vi "Module - MQTT Server.vi"(8 "error in (no error)":errorcluster) -> (0 "error out":errorcluster)   [LabVIEW 2020]
uses:
  Control/State - MQTT Server.ctl
  <vilib>/G Open Source Project for LabVIEW/MQTT Broker/Server class/Server.lvclass
  C:/Program Files (x86)/National Instruments/LabVIEW 2020/vi.lib/LabVIEW Open Source Project/MQTT Connection/MQTT_Base/Base Class/MQTT_Base.lvclass
  <vilib>/G Open Source Project for LabVIEW/MQTT Broker/Server class/Public Events -- cluster.ctl
  Shared/Control/State - eFGV.ctl
  Control/Config File Section List.ctl
  <vilib>/G Open Source Project for LabVIEW/MQTT Broker/Server class/Server.lvclass/Server.ctl
  <vilib>/LabVIEW Open Source Project/MQTT TCP Connection/MQTT_TCP/Connection/TCPConnection.lvclass
  C:/Program Files (x86)/National Instruments/LabVIEW 2020/vi.lib/LabVIEW Open Source Project/MQTT Connection/MQTT_Connection/Connection/Connection.lvclass
  <vilib>/LabVIEW Open Source Project/MQTT Connection/MQTT_Base/Base Class/MQTT_Base.lvclass
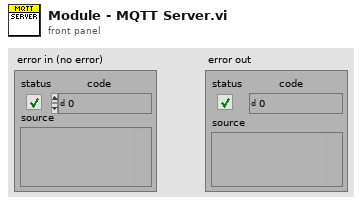
[diagram p1: front panel]
types:
  T1 = cluster{"MQTT Event":refnum<event-registration>, "User Event":refnum<event-registration>}
  T2 = cluster{"TOut":i32, "Module Name":string, "Server":refnum<class "Server.lvclass">, "User Exit":bool}
  T3 = typedef "State - MQTT Server.ctl" = enum16{"Init module", "Register for event", "Idle", "Create MQTT Broker", "Register MQTT Events", "Start MQTT Broker", "Re trigger MQTT Topic", "Stop MQTT Broker", "Unregister user event", "Close module"}
  T4 = typedef "State - eFGV.ctl" = enum16{"Init", "Read", "Write", "Close"}
  T5 = typedef "Config File Section List.ctl" = enum16{"sbRIO Setting", "RESTFUL Setting", "SQL Setting", "OPC Server Setting", "OPC Client Setting", "MQTT Server Setting", "MQTT Client Setting"}
  T6 = typedef "MQTT Server.lvlib/Server.lvclass/Public Events -- cluster.ctl" = cluster{"NbConnections":refnum<user-event>}
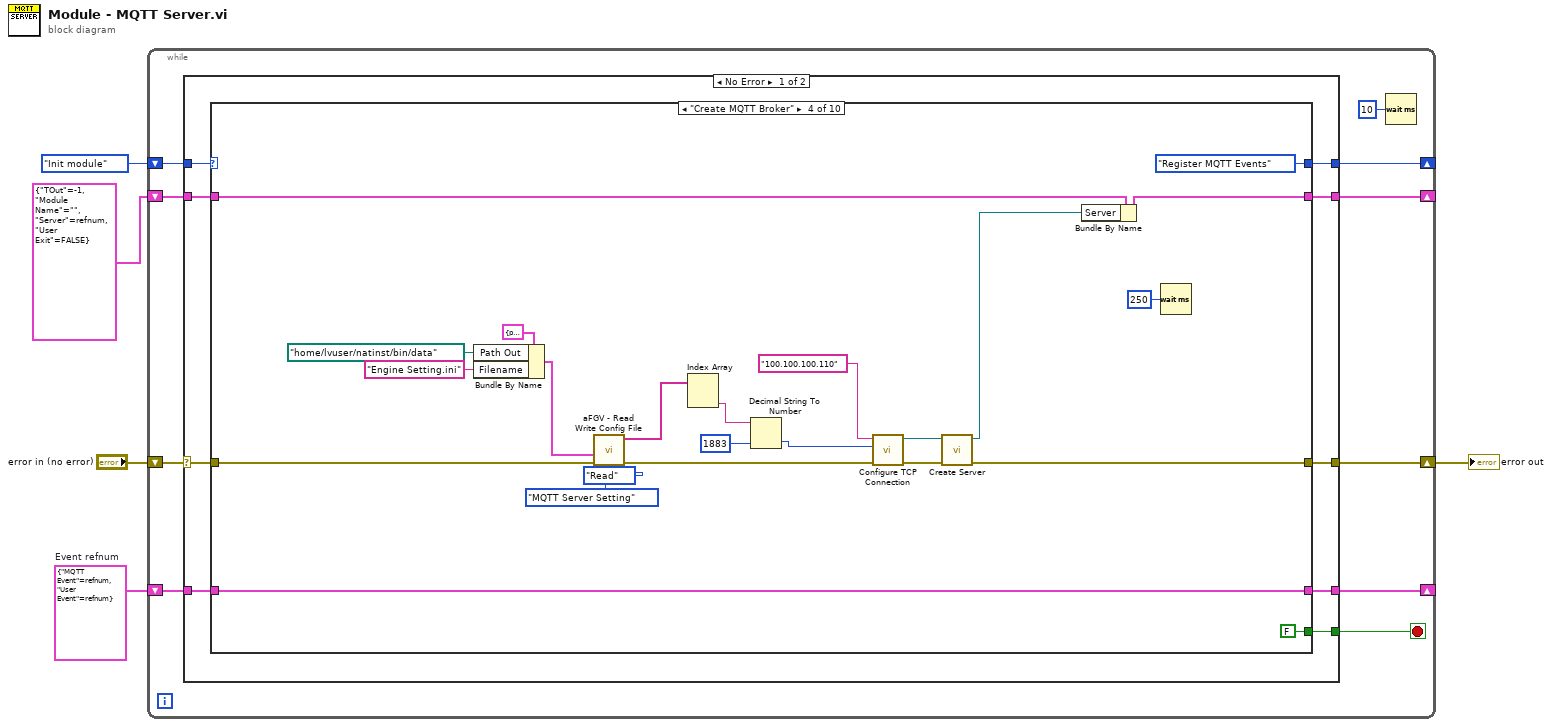
[diagram p0: block diagram]
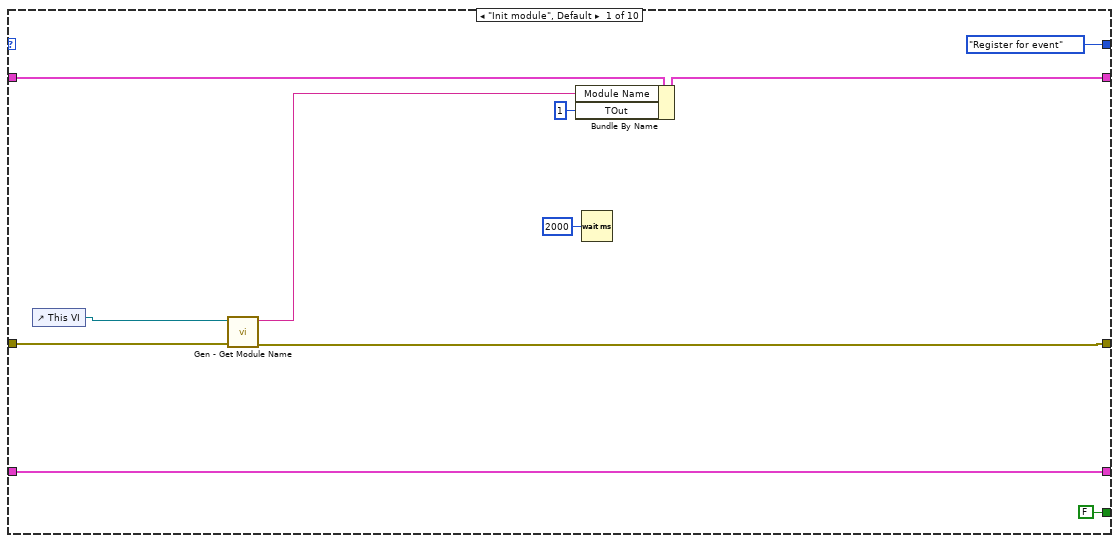
[diagram p2: hidden frame]
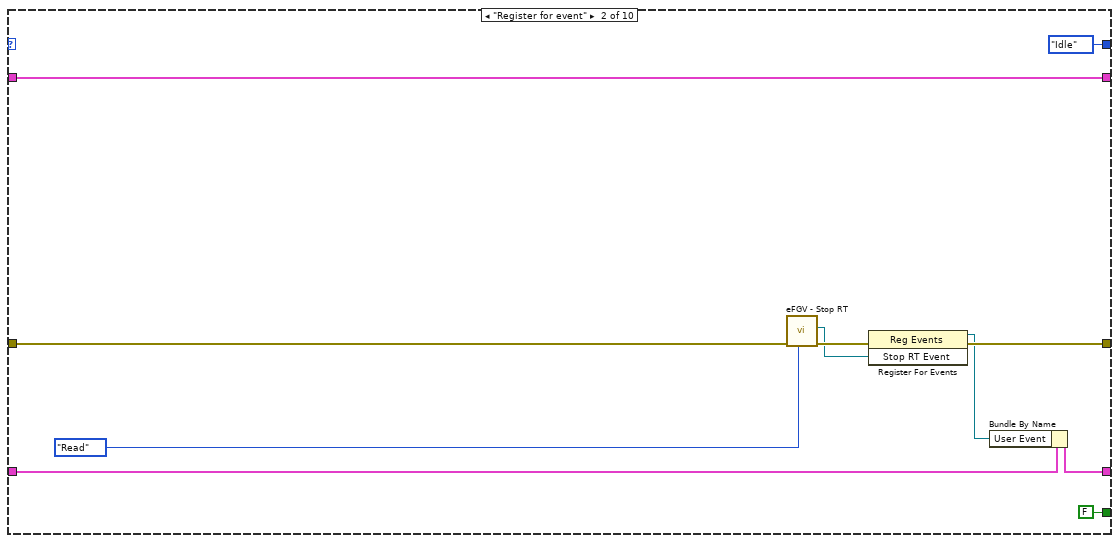
[diagram p3: hidden frame]
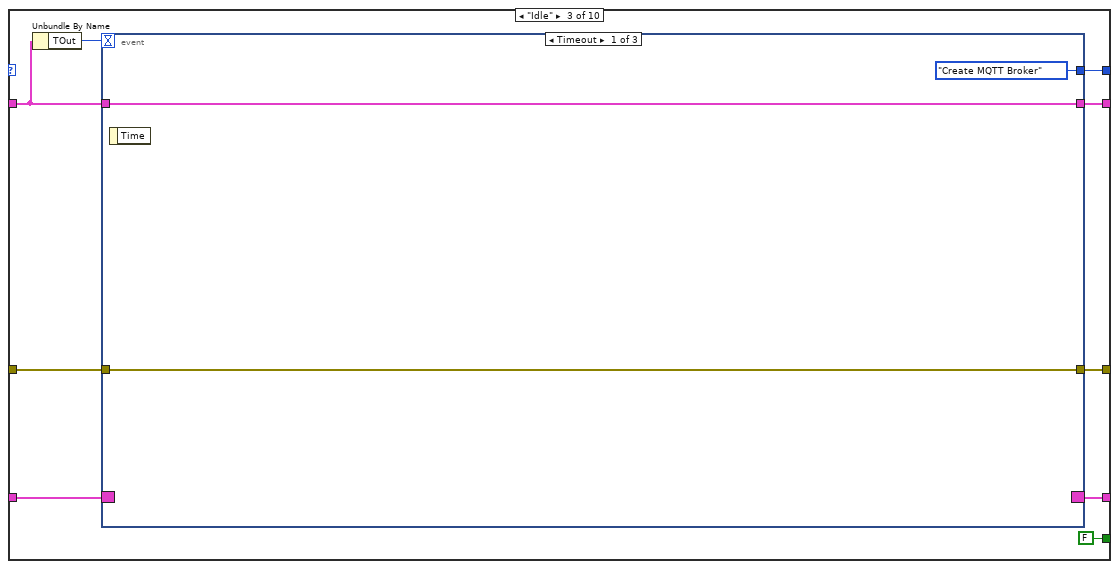
[diagram p4: hidden frame]
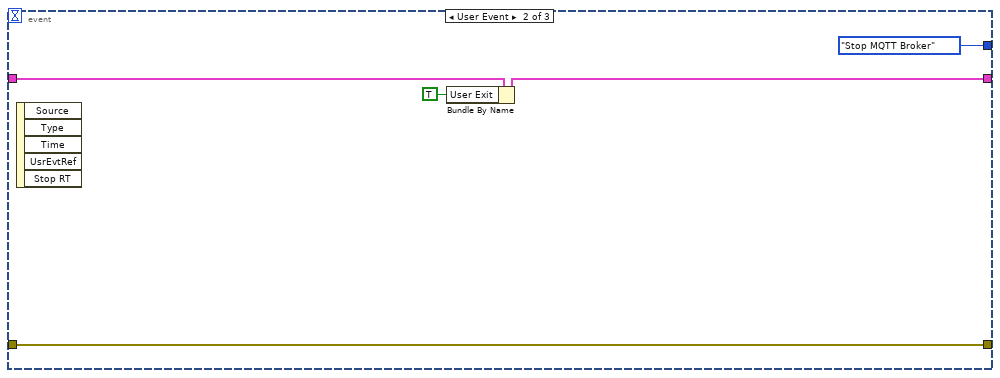
[diagram p5: hidden frame]
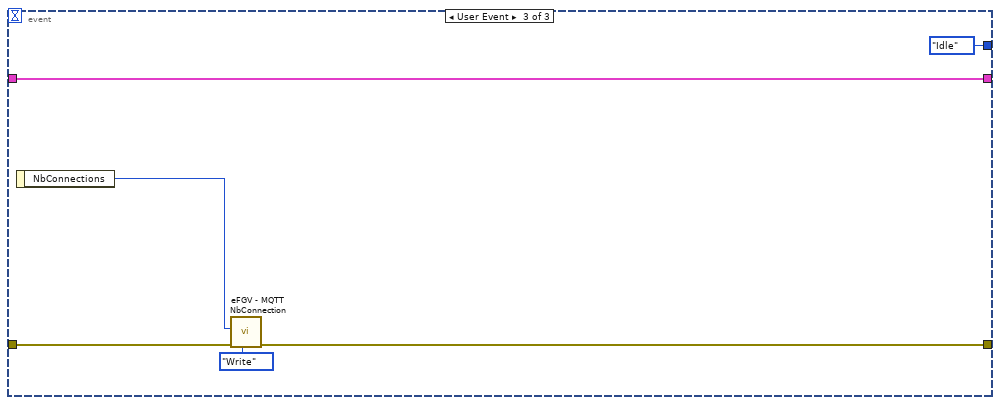
[diagram p6: hidden frame]
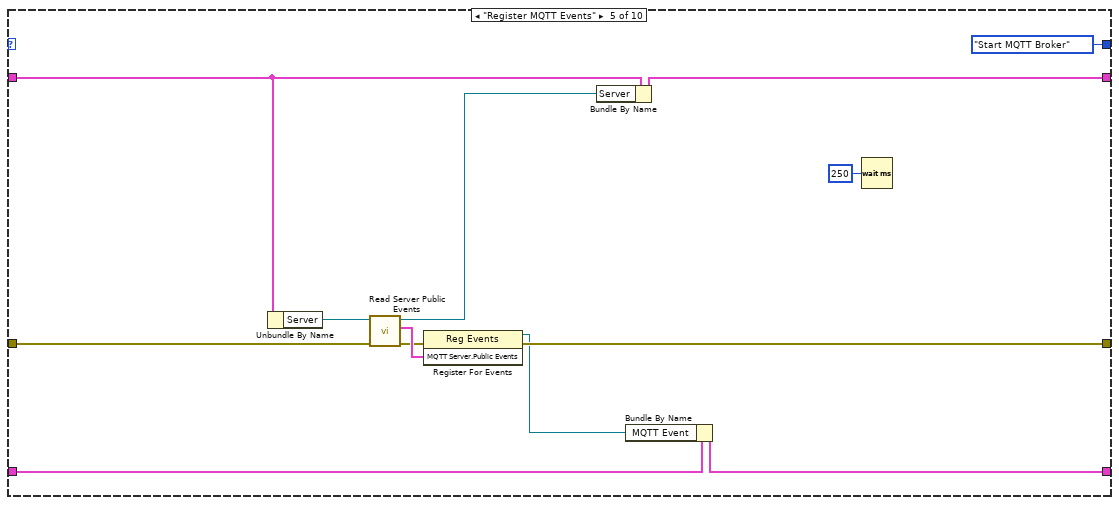
[diagram p7: hidden frame]
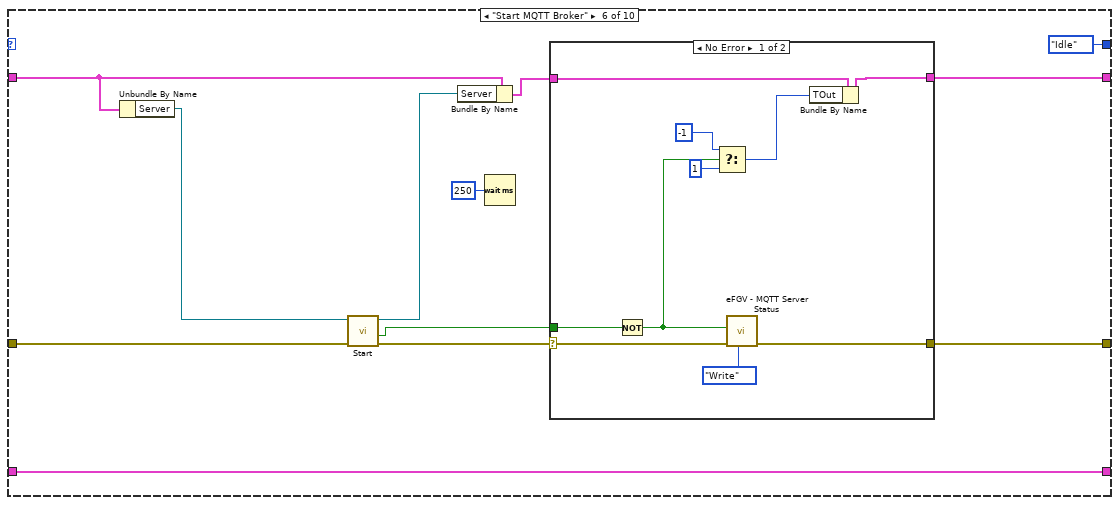
[diagram p8: hidden frame]
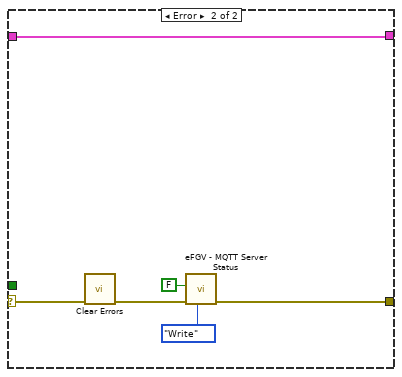
[diagram p9: hidden frame]
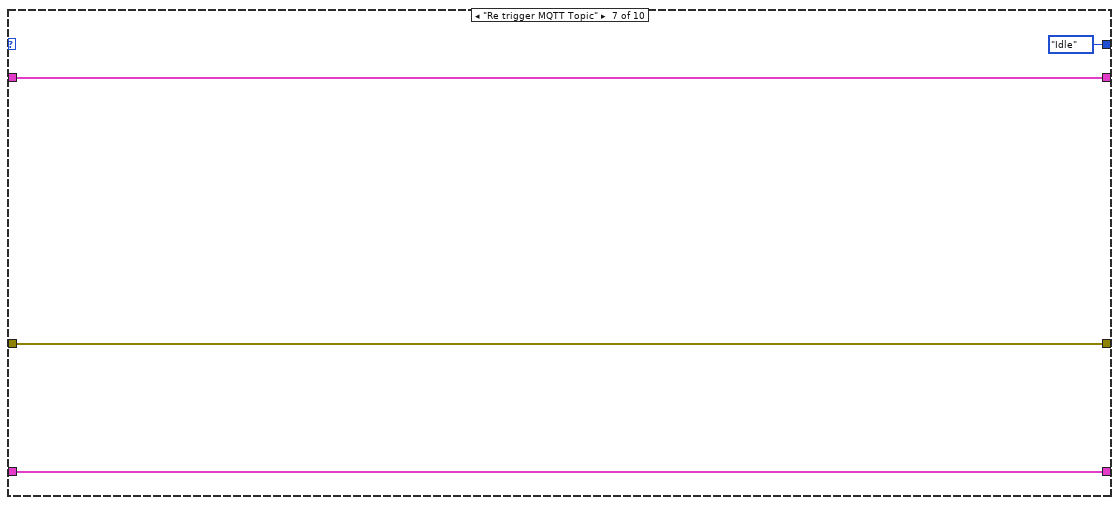
[diagram p10: hidden frame]
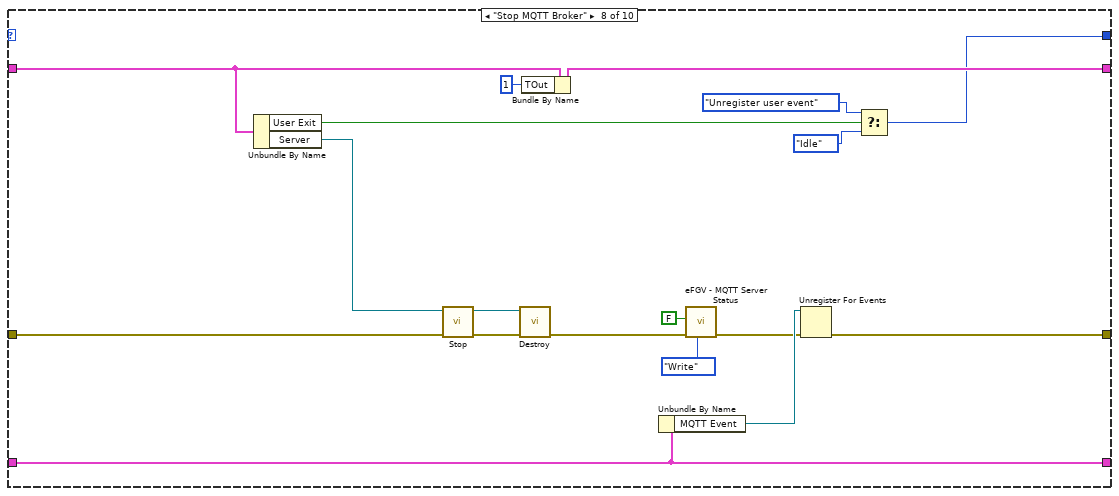
[diagram p11: hidden frame]
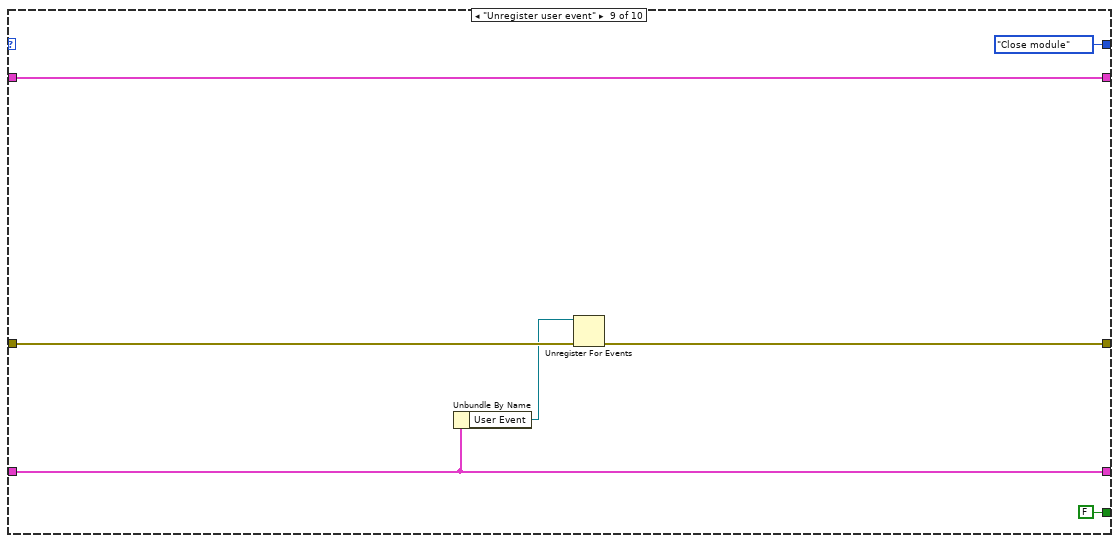
[diagram p12: hidden frame]
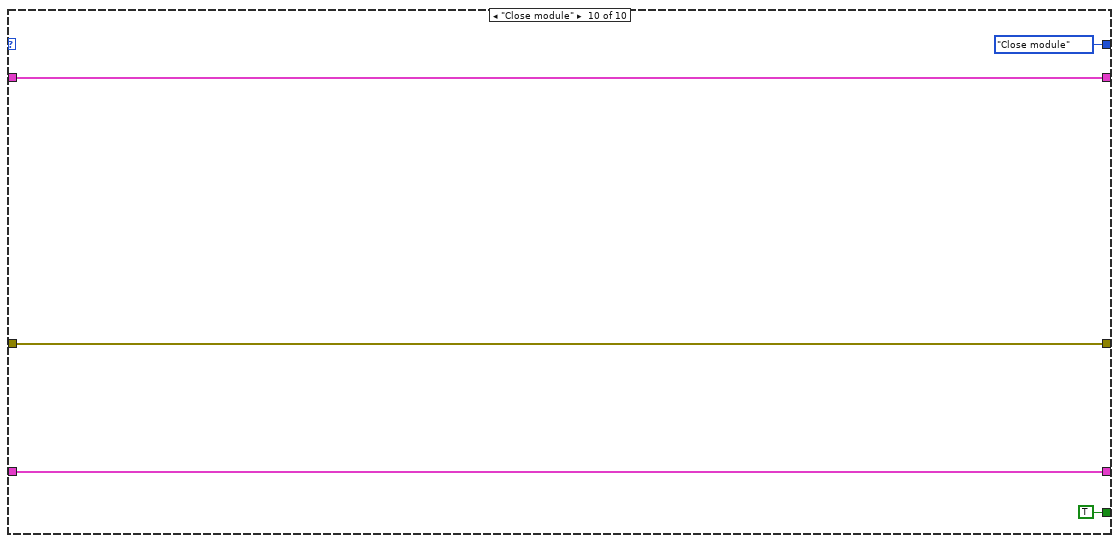
[diagram p13: hidden frame]
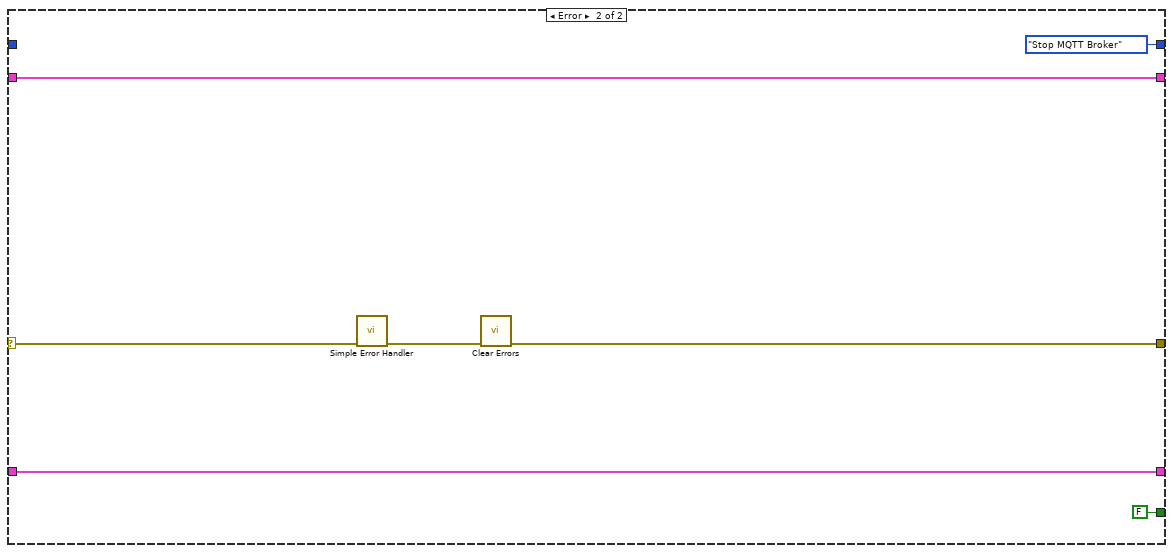
[diagram p14: hidden frame]
diagram:
  w1 = T1 {"MQTT Event"=refnum, "User Event"=refnum}  # Event refnum
  n1 = while {
    shift-right: [w11] -> w4
    shift-left: "error in (no error)" -> [w15]
    shift-right: [w7] -> _
    shift-left: State_-_MQTT_Server."Init module" -> [w13]
    shift-right: [w10] -> _
    shift-left: T2 {"TOut"=-1, "Module Name"="", "Server"=refnum, "User Exit"=FALSE} -> [w12]
    shift-right: [w8] -> _
    shift-left: w1 -> [w9]
    stop <- w14 stop-if-true
    n2 = case shown="No Error" w15 {
      selector: w15 -> [w24 w173]
      tunnel: [w23 FALSE] -> w14
      tunnel: w13 -> [w22 _]
      tunnel: w12 -> [w21 w170]
      tunnel: [w20 w171] -> w11
      tunnel: [w19 w170] -> w10
      tunnel: w9 -> [w18 w169]
      tunnel: [w17 w169] -> w8
      tunnel: [w16 State_-_MQTT_Server."Stop MQTT Broker"] -> w7
      frame No Error {
        n3 = case shown="\"Create MQTT Broker\"" w22 {
          tunnel: w24 -> [w32 w37 w55 w78 w103 w117 w137 w154 w161 w167]
          tunnel: [FALSE FALSE FALSE FALSE _ _ _ _ FALSE TRUE] -> w23
          tunnel: w21 -> [w34 w44 w52 w92 w100 w115 w136 w152 w162 w166]
          tunnel: [w31 w45 w54 w90 w102 w111 w137 w143 w160 w167] -> w20
          tunnel: [w30 w44 w51 w87 w96 w109 w136 w150 w162 w166] -> w19
          tunnel: w18 -> [w27 w41 w49 w85 w101 w116 w135 w144 w157 w164]
          tunnel: [w27 w40 w48 w85 w98 w116 w135 w144 w157 w164] -> w17
          tunnel: [State_-_MQTT_Server."Register for event" State_-_MQTT_Server."Idle" w47 State_-_MQTT_Server."Register MQTT Events" State_-_MQTT_Server."Start MQTT Broker" State_-_MQTT_Server."Idle" State_-_MQTT_Server."Idle" w145 State_-_MQTT_Server."Close module" State_-_MQTT_Server."Close module"] -> w16
          frame "Init module", Default {
            n4 = control-ref of="This VI"() -> (w33:refnum<vi>)
            n5 = call "Gen - Get Module Name.vi"("error in (no error)"=w32, "VI in"=w33) -> ("error out"=w31:errorcluster, "result string"=w29:string)  [unwired: 8 in]
            n6 = Bundle By Name(cluster=w34, "Module Name"=w29, "TOut"=1) -> (w30:T2)
            n7 = Wait (ms)(milliseconds to wait=u32 2000) -> ()  [unwired: 1 out]
          }
          frame "Register for event" {
            n8 = call "eFGV - Stop RT.vi"("State"=State_-_eFGV."Read", "error in (no error)"=w37) -> ("error out"=w43:errorcluster, "Stop RT Event"=w42:refnum<user-event>)  [unwired: 8 in]
            n9 = register-events(error in=w43, w42) -> (reference out=w39:refnum<event-registration>, error out=w45:errorcluster)  [unwired: 1 in]
            n10 = Bundle By Name(cluster=w41, "User Event"=w39) -> (w40:T1)
          }
          frame "Idle" {
            n11 = Unbundle By Name(w52) -> ("TOut"=w53:i32)
            n12 = event shown="[0] Timeout" {
              selector: w49 -> [_ _ _]
              dyn-events: [_ _ _] -> w48
              timeout: w53 -> [_ _ _]
              tunnel: w55 -> [w58 w62 w67]
              tunnel: [w58 w62 w66] -> w54
              tunnel: w52 -> [w57 w63 w68]
              tunnel: [w57 w60 w68] -> w51
              tunnel: [State_-_MQTT_Server."Create MQTT Broker" State_-_MQTT_Server."Stop MQTT Broker" State_-_MQTT_Server."Idle"] -> w47
              event Timeout {
                n13 = event-data() -> ()  [unwired: 1 in, 1 out]
              }
              event User Event {
                n14 = event-data() -> ()  [unwired: 1 in, 5 out]
                n15 = Bundle By Name(cluster=w63, "User Exit"=TRUE) -> (w60:T2)
              }
              event User Event {
                n16 = event-data() -> ("NbConnections"=w65:u32)  [unwired: 1 in]
                n17 = call "eFGV - MQTT NbConnection.vi"("State"=State_-_eFGV."Write", "error in (no error)"=w67, "NbConnections"=w65) -> ("error out"=w66:errorcluster)  [unwired: 7 in, 1 out]
              }
            }
          }
          frame "Create MQTT Broker" {
            n18 = Bundle By Name(cluster=cluster{"Path Out":path, "Filename":string} {"Path Out"=path "", "Filename"=""} ("Path File"), "Path Out"=path "/home/lvuser/natinst/bin/data" ("appended path"), "Filename"="Engine Setting.ini") -> (w84:cluster{"Path Out":path, "Filename":string})
            n19 = call "aFGV - Read Write Config File.vi"("State"=enum16{"Read", "Write", "Delete"}."Read", "Section"=Config_File_Section_List."MQTT Server Setting", "Error In"=w78, "Path File"=w84) -> ("Error Out"=w77:errorcluster, "Data out"=w76:string[])  [unwired: 5 in, 1 out]
            n20 = Index Array(array=w76) -> (element #2=w74:string)  [unwired: 2 in, 1 out]
            n21 = Decimal String To Number(string=w74, default (0L)=u16 1883 ("remote port (80)")) -> (number=w73:u16)  [unwired: 1 in, 1 out]
            n22 = call <vilib>:"Configure TCP Connection.vi"("error in (no error)"=w77, "remote port (80)"=w73, "address (localhost)"="100.100.100.110") -> ("error out"=w89:errorcluster, "TCPConnection"=w88:refnum<class "TCPConnection.lvclass">)  [unwired: 7 in]
            n23 = call <vilib>:"Create Server.vi"("error in (no error)"=w89, "Connection Configuration"=w88) -> ("error out"=w90:errorcluster, "Server"=w86:refnum<class "Server.lvclass">)  [unwired: 8 in]
            n24 = Bundle By Name(cluster=w92, "Server"=w86) -> (w87:T2)
            n25 = Wait (ms)(milliseconds to wait=u32 250) -> ()  [unwired: 1 out]
          }
          frame "Register MQTT Events" {
            n26 = Unbundle By Name(w100) -> ("Server"=w99:refnum<class "Server.lvclass">)
            n27 = call <vilib>:"Read Server Public Events.vi"("error in (no error)"=w103, "Server in"=w99) -> ("error out"=w104:errorcluster, "MQTT Server.Public Events"=w105:T6, "Server out"=w95:refnum<class "Server.lvclass">)  [unwired: 7 in]
            n28 = register-events(error in=w104, w105) -> (reference out=w97:refnum<event-registration>, error out=w102:errorcluster)  [unwired: 1 in]
            n29 = Bundle By Name(cluster=w100, "Server"=w95) -> (w96:T2)
            n30 = Bundle By Name(cluster=w101, "MQTT Event"=w97) -> (w98:T1)
            n31 = Wait (ms)(milliseconds to wait=u32 250) -> ()  [unwired: 1 out]
          }
          frame "Start MQTT Broker" {
            n32 = Unbundle By Name(w115) -> ("Server"=w114:refnum<class "Server.lvclass">)
            n33 = call <vilib>:"Start.vi"("error in (no error)"=w117, "MQTT_Base in"=w114) -> ("error out"=w112:errorcluster, "timed out?"=w110:bool, "MQTT_Base out"=w113:refnum<class "Server.lvclass">)  [unwired: 7 in]
            n34 = Bundle By Name(cluster=w115, "Server"=w113) -> (w108:T2)
            n35 = Wait (ms)(milliseconds to wait=u32 250) -> ()  [unwired: 1 out]
            n36 = case shown="No Error" w112 {
              selector: w112 -> [w120 w133]
              tunnel: [w119 w130] -> w111
              tunnel: w110 -> [w127 _]
              tunnel: [w125 w132] -> w109
              tunnel: w108 -> [w126 w132]
              frame No Error {
                n37 = Not(x=w127) -> (.not. x?=w118:bool)
                n38 = Select(t=-1 ("TOut"), s=w118, f=1) -> (s? t:f=w122:i32)
                n39 = call "eFGV - MQTT Server Status.vi"("State"=State_-_eFGV."Write", "error in (no error)"=w120, "MQTT Server Created"=w118) -> ("error out"=w119:errorcluster)  [unwired: 7 in, 1 out]
                n40 = Bundle By Name(cluster=w126, "TOut"=w122) -> (w125:T2)
              }
              frame Error {
                n41 = call <vilib>:"Clear Errors.vi"("error in (no error)"=w133) -> ("error out"=w131:errorcluster)  [unwired: 5 in, 1 out]
                n42 = call "eFGV - MQTT Server Status.vi"("State"=State_-_eFGV."Write", "error in (no error)"=w131, "MQTT Server Created"=FALSE) -> ("error out"=w130:errorcluster)  [unwired: 7 in, 1 out]
              }
            }
          }
          frame "Re trigger MQTT Topic" {
          }
          frame "Stop MQTT Broker" {
            n43 = Unbundle By Name(w152) -> ("User Exit"=w148:bool, "Server"=w151:refnum<class "Server.lvclass">)
            n44 = call <vilib>:"Stop.vi"("error in (no error)"=w154, "MQTT_Base in"=w151) -> ("error out"=w155:errorcluster, "MQTT_Base out"=w153:refnum<class "Server.lvclass">)  [unwired: 7 in, 1 out]
            n45 = call <vilib>:"Destroy.vi"("error in (no error)"=w155, "MQTT_Base in"=w153) -> ("error out"=w139:errorcluster)  [unwired: 8 in, 1 out]
            n46 = Bundle By Name(cluster=w152, "TOut"=1) -> (w150:T2)
            n47 = Unbundle By Name(w144) -> ("MQTT Event"=w142:refnum<event-registration>)
            n48 = call "eFGV - MQTT Server Status.vi"("State"=State_-_eFGV."Write", "error in (no error)"=w139, "MQTT Server Created"=FALSE) -> ("error out"=w138:errorcluster)  [unwired: 7 in, 1 out]
            n49 = Unregister For Events(event registration refnum=w142, error in=w138) -> (error out=w143:errorcluster)
            n50 = Select(t=State_-_MQTT_Server."Unregister user event", s=w148, f=State_-_MQTT_Server."Idle") -> (s? t:f=w145:T3)
          }
          frame "Unregister user event" {
            n51 = Unbundle By Name(w157) -> ("User Event"=w156:refnum<event-registration>)
            n52 = Unregister For Events(event registration refnum=w156, error in=w161) -> (error out=w160:errorcluster)
          }
          frame "Close module" {
          }
        }
      }
      frame Error {
        n53 = call <vilib>:"Simple Error Handler.vi"("error in (no error)"=w173) -> ("error out"=w172:errorcluster)  [unwired: 4 in, 4 out]
        n54 = call <vilib>:"Clear Errors.vi"("error in (no error)"=w172) -> ("error out"=w171:errorcluster)  [unwired: 5 in, 1 out]
      }
    }
    n55 = Wait (ms)(milliseconds to wait=u32 10) -> ()  [unwired: 1 out]
  }
  "error out" <- w4
